vi "CRYGet Device Informaion.vi"(11 "error in (no error)":errorcluster) -> (4 "Output Device Infor":T1(array[cluster]), 6 "Output Device Name":string[](array[string]), 8 "Input Device Infor":T1(array[cluster]), 10 "Input Device Name":string[](array[string]), 15 "error out":errorcluster)   [LabVIEW 2013]
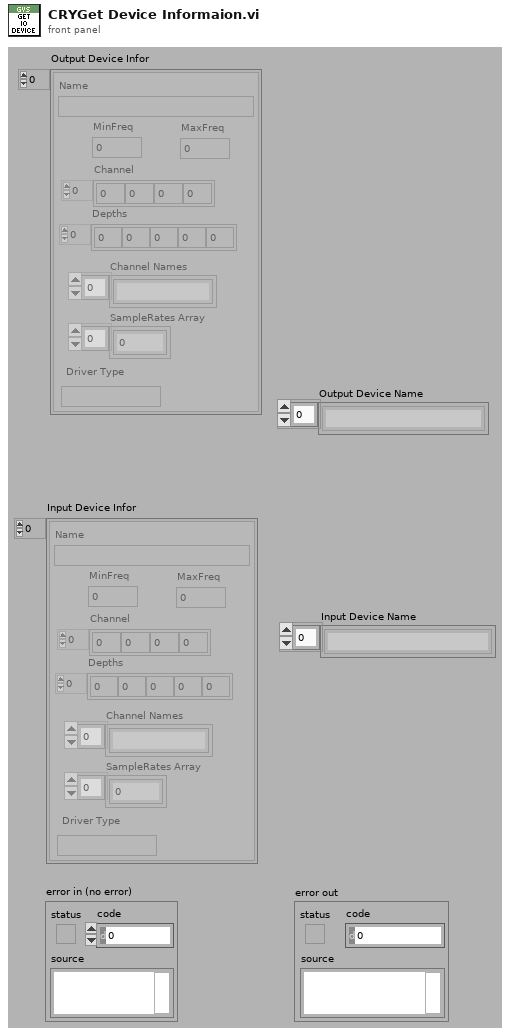
[diagram p1: front panel]
types:
  T1 = cluster{"Name":string, "MinFreq":dbl, "MaxFreq":dbl, "Channel":i32[], "Depths":i32[], "Channel Names":string[], "SampleRates Array":dbl[], "Driver Type":string}[]
  T2 = cluster{"Name":string, "MinFreq":dbl, "MaxFreq":dbl, "Channel":i32[], "Depths":i32[], "Channel Names":string[], "SampleRates Array":dbl[], "Driver Type":string}
  T3 = cluster{"channels":i32[], "depths":i32[], "minFreq":dbl, "maxFreq":dbl}
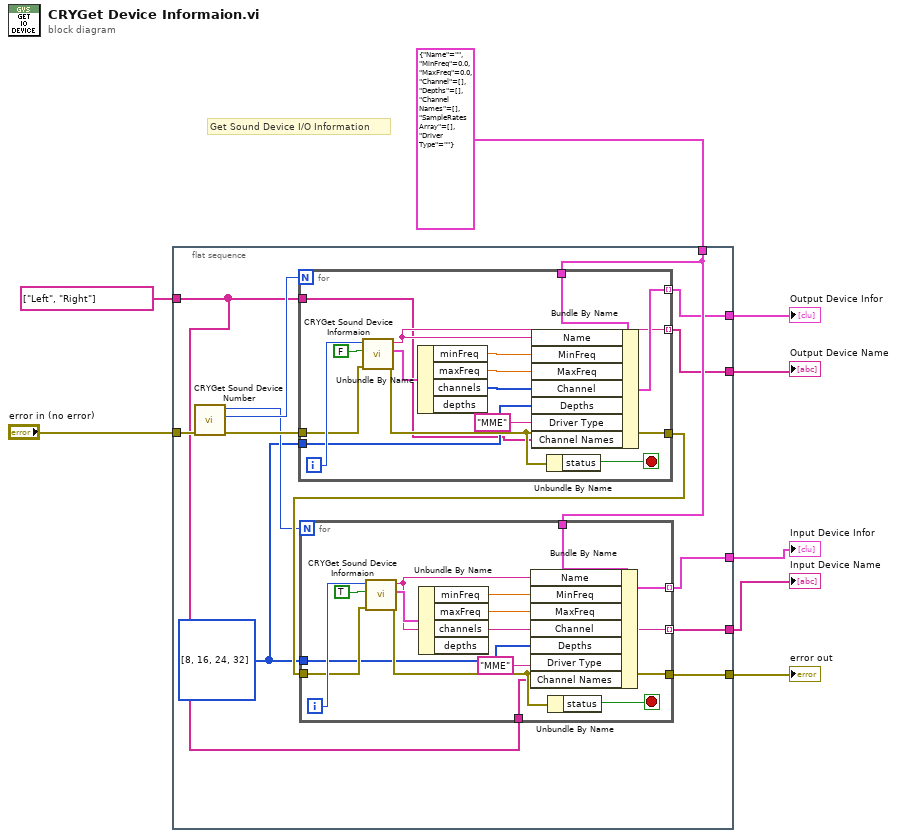
[diagram p0: block diagram]
diagram:
  # "Get Sound Device I/O Information"
  n1 = flat-sequence {
    tunnel: "error in (no error)" -> [w21]
    tunnel: T2 {"Name"="", "MinFreq"=0.0, "MaxFreq"=0.0, "Channel"=[], "Depths"=[], "Channel Names"=[], "SampleRates Array"=[], "Driver Type"=""} ("I_Device Infor") -> [w16]
    tunnel: [w15] -> w6
    tunnel: [w14] -> w5
    tunnel: [w13] -> w4
    tunnel: [w12] -> w3
    tunnel: [w11] -> w2
    tunnel: string[] ["Left", "Right"] -> [w9]
    frame #0 {
      w10 = i32[] [8, 16, 24, 32] ("Depths")
      n2 = call "CRYGet Sound Device Number.vi"("error in (no error)"=w21) -> ("error out"=w19:errorcluster, "Number of Output Devices"=w18:i32, "Number of Input Devices"=w17:i32)  [unwired: 8 out]
      n3 = for {
        N: w18 -> [_]
        tunnel: w19 -> [w46]
        tunnel: [w45] -> w20
        tunnel: w16 -> [w43]
        tunnel: w10 -> [w41]
        tunnel: [w40] -> w15 mode=indexing
        tunnel: [w39] -> w14 mode=indexing
        tunnel: w9 -> [w37]
        i -> [w51]
        stop <- w44 stop-if-true
        n4 = call "CRYGet Sound Device Informaion.vi"("error in (no error)"=w46, "isInput?"=FALSE, "device"=w51) -> ("error out"=w45:errorcluster, "Capabilities"=w50:T3, "Device Name"=w39:string)  [unwired: 6 out]
        n5 = Unbundle By Name(w50) -> ("minFreq"=w49:dbl, "maxFreq"=w48:dbl, "channels"=w47:i32[])  [unwired: 1 out]
        n6 = Bundle By Name(cluster=w43, "Name"=w39, "MinFreq"=w49, "MaxFreq"=w48, "Channel"=w47, "Depths"=w41, "Driver Type"="MME", "Channel Names"=w37) -> (w40:T2)
        n7 = Unbundle By Name(w45) -> ("status"=w44:bool)
      }
      n8 = for {
        N: w17 -> [_]
        tunnel: w20 -> [w32]
        tunnel: [w31] -> w11
        tunnel: w16 -> [w29]
        tunnel: w10 -> [w27]
        tunnel: [w26] -> w13 mode=indexing
        tunnel: [w25] -> w12 mode=indexing
        tunnel: w9 -> [w23]
        i -> [w36]
        stop <- w30 stop-if-true
        n9 = call "CRYGet Sound Device Informaion.vi"("error in (no error)"=w32, "isInput?"=TRUE, "device"=w36) -> ("error out"=w31:errorcluster, "Capabilities"=w35:T3, "Device Name"=w25:string)  [unwired: 6 out]
        n10 = Unbundle By Name(w35) -> ("minFreq"=w34:dbl, "maxFreq"=w33:dbl, "channels"=w22:i32[])  [unwired: 1 out]
        n11 = Bundle By Name(cluster=w29, "Name"=w25, "MinFreq"=w34, "MaxFreq"=w33, "Channel"=w22, "Depths"=w27, "Driver Type"="MME", "Channel Names"=w23) -> (w26:T2)
        n12 = Unbundle By Name(w31) -> ("status"=w30:bool)
      }
    }
  }
  "Output Device Infor" <- w6
  "Input Device Infor" <- w4
  "error out" <- w2
  "Output Device Name" <- w5
  "Input Device Name" <- w3
